vi "Energy.vi"   [LabVIEW 2013, in "NI_EP_Basic.lvlib"]
doc: "Calculates the energy value from the power value for a specified interval. This VI returns the value of active energy, apparent energy, and reactive energy. Wire data to the <B>power value</B> input to determine the polymorphic instance to use or manually select the instance."
uses:
  <vilib>/addons/Electrical Power/Basic/NI_EP_Basic.lvlib
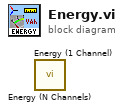
[diagram p0: block diagram]
diagram:
  n1 = call <vilib>:"Energy (N Channels).vi"() -> ()  [unwired: 9 in, 3 out]
  n2 = call <vilib>:"Energy (1 Channel).vi"() -> ()  [unwired: 9 in, 3 out]
